vi "To File (Path).vi"(6 "enable LabVIEW extensions? (T)":bool=TRUE, 7 "Pretty Print?":bool=TRUE, 8 "error in (no error)":errorcluster, 10 "Variant in":variant, 11 "path in":path) -> (0 "error out":errorcluster, 3 "path out":path)   [LabVIEW 2017, in "Variant JSON API.lvlib"]
doc: "Saves a JSON instance's data to the given file."
uses:
  Variant JSON API.lvlib
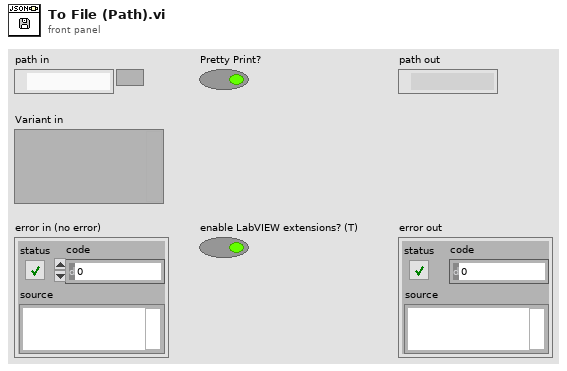
[diagram p1: front panel]
types:
  T1 = enum16{"open", "replace", "create", "open or create", "replace or create", "replace or create with confirmation"}
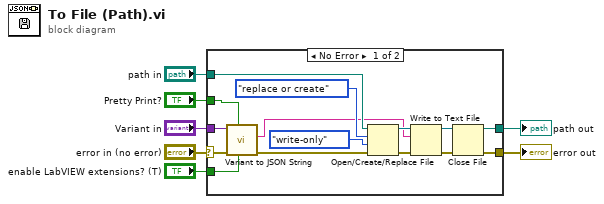
[diagram p0: block diagram]
diagram:
  n1 = case shown="No Error" "error in (no error)" {
    selector: "error in (no error)" -> [w18 w24]
    tunnel: "Variant in" -> [w22 _]
    tunnel: "path in" -> [w16 w23]
    tunnel: [w15 w24] -> w4
    tunnel: "Pretty Print?" -> [w10 _]
    tunnel: "enable LabVIEW extensions? (T)" -> [w9 _]
    tunnel: [w12 w23] -> w1
    frame No Error {
      n2 = call "Variant to JSON String.vi"("enable LabVIEW extensions? (T)"=w9, "pretty print? (F)"=w10, "error in (no error)"=w18, "Variant in"=w22) -> ("error out"=w14:errorcluster, "String"=w8:string)  [unwired: 5 in, 1 out]
      n3 = Open/Create/Replace File(file path (use dialog)=w16, error in=w14, operation (0:open)=T1."replace or create", access (0:read/write)=enum16{"read/write", "read-only", "write-only"}."write-only") -> (refnum out=w19:refnum<file>, error out=w17:errorcluster)  [unwired: 2 in, 1 out]
      n4 = Write to Text File(file (use dialog)=w19, text=w8, error in=w17) -> (refnum out=w20:refnum<file>, error out=w21:errorcluster)  [unwired: 1 in, 1 out]
      n5 = Close File(refnum=w20, error in=w21) -> (path=w12:path, error out=w15:errorcluster)
    }
    frame Error {
    }
  }
  "error out" <- w4
  "path out" <- w1
